vi "Current Position Write.vi"(4 "error in (no error)":errorcluster, 5 "Value":i32, 6 "Container State":T2, 7 "Display State In":T1) -> (0 "error out":errorcluster, 3 "Display State Out":T1)   [LabVIEW 2012, in "Waveform Control.xctl"]
uses:
  Waveform Control.xctl
  <vilib>/_xctls/Container State.ctl
  Controls/State.ctl
  Controls/Volatile State Ops.ctl
  <vilib>/_xctls/XControlSupport.lvlib
panel:
  # "Replace the Value Control below with a Control of desired type.\nDo not remove this Control or the others from the connector pane.\nDo not change the connector pane pattern.\nThe Value control should always be the third terminal from top on the input side in the connector pane."
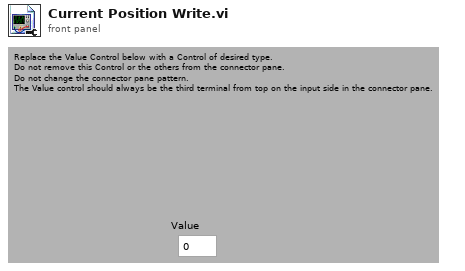
[diagram p1: front panel]
types:
  T1 = typedef "Waveform Control.xctl/State.ctl" = cluster{"Name":string}
  T2 = typedef "XControlSupport.lvlib/Container State.ctl" = cluster{"Indicator?":bool, "Run Mode?":bool, " Refnum":refnum<vi>}
  T3 = typedef "Waveform Control.xctl/Volatile State Ops.ctl" = enum16{"Read", "Write", "Update State from Data"}
  T4 = typedef "Waveform Control.xctl/Waveform State.ctl" = cluster{"Show Axes":bool, "Show Y=0":bool, "Controls":T5, "Show Current Location":bool, "Current Location":i32, "dt":dbl, "t0":timestamp, "Format and Units":string}
  T5 = typedef "Waveform Control.xctl/FP Controls.ctl" = cluster{"Type":T6, "Periods":dbl, "Points":i32, "Offset":dbl, "Amplitdue":dbl, "Phase":dbl, "func":string}
  T6 = typedef "Waveform Control.xctl/Function Types.ctl" = enum16{"Level", "Sine", "Triangle", "Ramp", "Saw Tooth", "Square", "Function"}
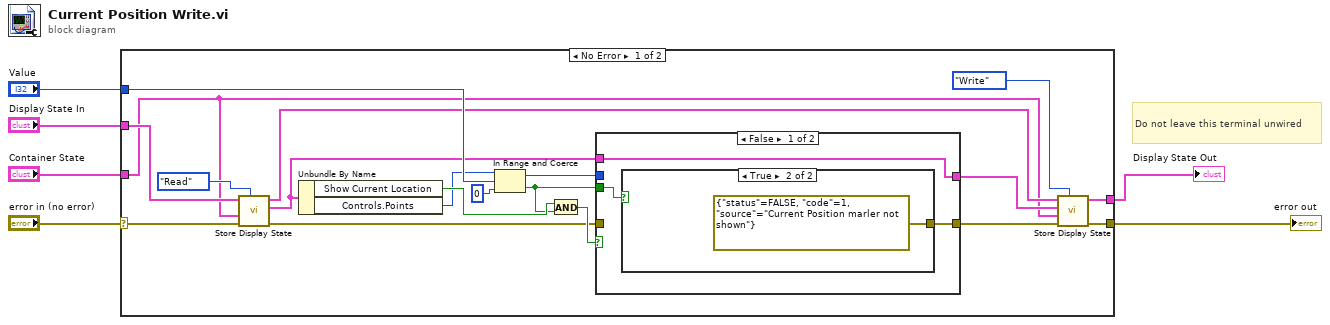
[diagram p0: block diagram]
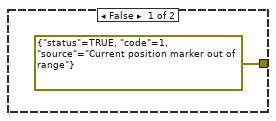
[diagram p2: hidden frame]
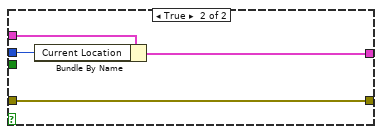
[diagram p3: hidden frame]
diagram:
  # "Do not leave this terminal unwired"
  n1 = case shown="No Error" "error in (no error)" {
    selector: "error in (no error)" -> [w18 w36]
    tunnel: "Value" -> [w24 _]
    tunnel: [w9 w35] -> w5
    tunnel: [w12 w36] -> w4
    tunnel: "Display State In" -> [w16 w35]
    tunnel: "Container State" -> [w7 _]
    frame No Error {
      n2 = call "Store Display State.vi"("Operation In"=Volatile_State_Ops."Read", "Error In (no Error) In"=w18, "Container State In"=w7, "State In"=w16) -> ("Error Out"=w17:errorcluster, "Waveform State Out"=w15:T4, "Display State Out"=w10:T1)  [unwired: 2 in, 3 out]
      n3 = Unbundle By Name(w15) -> ("Show Current Location"=w25:bool, "Controls.Points"=w19:i32)
      n4 = In Range and Coerce(upper limit=w19, x=w24, lower limit=0) -> (coerced(x)=w22:i32, In Range?=w20:bool)
      n5 = And(x=w25, y=w20) -> (x .and. y?=w21:bool)
      n6 = case shown="False" w21 {
        tunnel: w15 -> [w28 w34]
        tunnel: w22 -> [_ w33]
        tunnel: [w28 w32] -> w11
        tunnel: w17 -> [_ w31]
        tunnel: [w26 w31] -> w13
        tunnel: w20 -> [w27 _]
        frame False {
          n7 = case shown="True" w27 {
            tunnel: [errorcluster {"status"=TRUE, "code"=1, "source"="Current position marker out of range"} ("error IO") errorcluster {"status"=FALSE, "code"=1, "source"="Current Position marler not shown"} ("error IO")] -> w26
            frame False {
            }
            frame True {
            }
          }
        }
        frame True {
          n8 = Bundle By Name(cluster=w34, "Current Location"=w33) -> (w32:T4)
        }
      }
      n9 = call "Store Display State.vi"("Operation In"=Volatile_State_Ops."Write", "Error In (no Error) In"=w13, "Container State In"=w7, "Waveform State In"=w11, "State In"=w10) -> ("Error Out"=w12:errorcluster, "Display State Out"=w9:T1)  [unwired: 1 in, 4 out]
    }
    frame Error {
    }
  }
  "error out" <- w4
  "Display State Out" <- w5
